vi "Make Switch Enumeration.vi"(7 "State (0: ssNone)":i32(ring) items=["ssNone", "ssA", "ssB"], 8 "error in (no error)":errorcluster, 9 "Channel Enum (0)":i32, 10 "Switch Type (0: stBNCOutput)":i32(ring) items=["stBNCOutput", "stBNCInput", "stXLROutput", "stXLRInput"], 11 "VISA resource name":refnum<visa-resource-name>) -> (0 "error out":errorcluster, 3 "VISA resource name out":refnum<visa-resource-name>)   [LabVIEW 2014, in "Stanford Research SR1.lvlib"]
doc: "Connects the logical channel of the specified network to either A,B, or nothing (disconnected)."
uses:
  Stanford Research SR1.lvlib
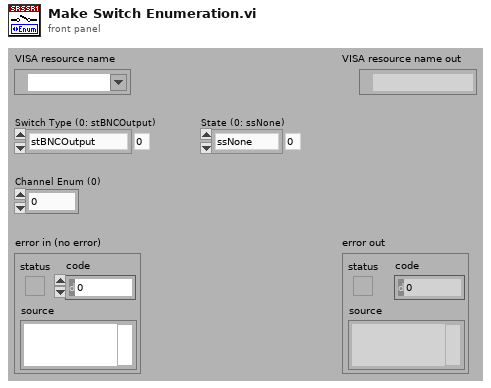
[diagram p1: front panel]
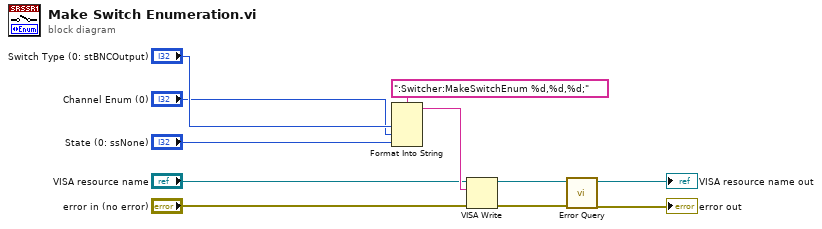
[diagram p0: block diagram]
diagram:
  n1 = Format Into String(format string=":Switcher:MakeSwitchEnum %d,%d,%d;", "Switch Type (0: stBNCOutput)", "Channel Enum (0)", "State (0: ssNone)") -> (resulting string=w7:string)  [unwired: 2 in, 1 out]
  n2 = VISA Write(VISA resource name="VISA resource name", write buffer=w7, error in (no error)="error in (no error)") -> (VISA resource name out=w4:refnum<visa-resource-name>, error out=w3:errorcluster)  [unwired: 1 out]
  n3 = call "Error Query.vi"("error in (no error)"=w3, "VISA resource name"=w4) -> ("error out"=→"error out":errorcluster, "VISA resource name out"=→"VISA resource name out":refnum<visa-resource-name>)  [unwired: 6 in, 2 out]
